vi "delete_scope_data_Qs.vi"(7 "scope Q data":T1) -> (8 "error out":errorcluster)   [LabVIEW 2023]
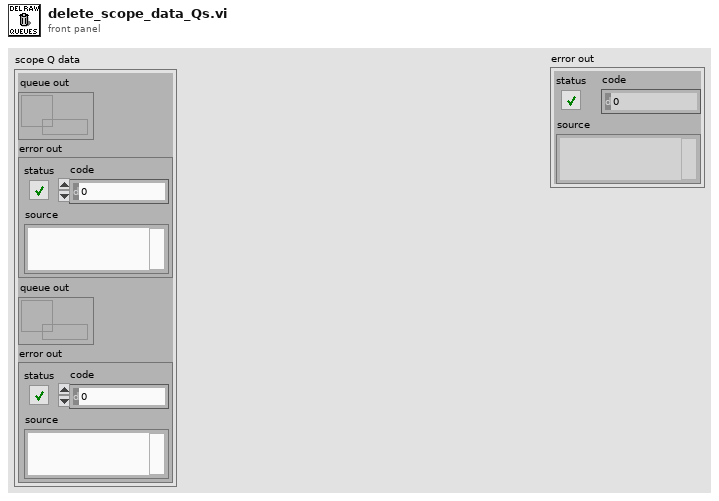
[diagram p1: front panel]
types:
  T1 = cluster{"queue out":refnum<queue>, "error out":errorcluster, "queue out":refnum<queue>, "error out":errorcluster}
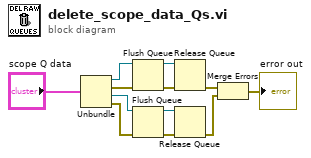
[diagram p0: block diagram]
diagram:
  n1 = Unbundle("scope Q data") -> ("queue out"=w8:refnum<queue>, "error out"=w7:errorcluster, "queue out"=w6:refnum<queue>, "error out"=w5:errorcluster)
  n2 = Flush Queue(queue=w8, error in (no error)=w7) -> (queue out=w12:refnum<queue>, error out=w11:errorcluster)  [unwired: 1 out]
  n3 = Flush Queue(queue=w6, error in (no error)=w5) -> (queue out=w10:refnum<queue>, error out=w9:errorcluster)  [unwired: 1 out]
  n4 = Release Queue(queue=w12, error in (no error)=w11) -> (error out=w4:errorcluster)  [unwired: 1 in, 2 out]
  n5 = Release Queue(queue=w10, error in (no error)=w9) -> (error out=w3:errorcluster)  [unwired: 1 in, 2 out]
  n6 = Merge Errors(w4, w3) -> (→"error out":errorcluster)
